vi "tutorial 7.vi"() -> ()   [LabVIEW 2022 SP3]
panel:
  out "return value":cluster{string, string, string}[](array[cluster])
  in  "user input":string
  in  "stop":bool
  in  "function name":string
  in  "Python version":string
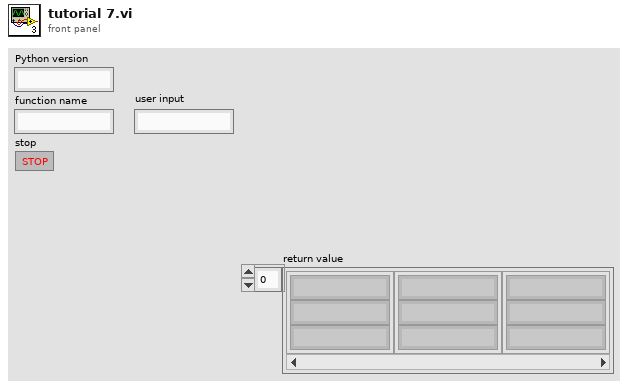
[diagram p1: front panel]
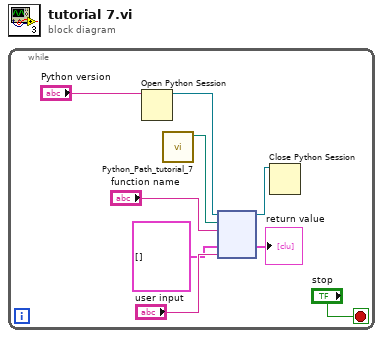
[diagram p0: block diagram]
diagram:
  n1 = while {
    stop <- "stop" stop-if-true
    n2 = Open Python Session(python version="Python version") -> (session out=w6:refnum<k35>)  [unwired: 2 in, 1 out]
    n3 = call "Python_Path_tutorial_7.vi"() -> ("appended path"=w7:path)  [unwired: 11 in]
    n4 = node(w6, w7, "function name", cluster{string, string, string}[] [], "user input") -> (w8:refnum<k35>, →"return value":cluster{string, string, string}[])  [unwired: 2 in, 3 out]
    n5 = Close Python Session(session in=w8) -> ()  [unwired: 1 in, 1 out]
  }
